vi "Send single trigger.vi"(8 "error in (no error)":errorcluster, 11 "SA-ESA in":refnum<class "SA-ESA.lvclass">) -> (0 "error out":errorcluster, 3 "SA-ESA out":refnum<class "SA-ESA.lvclass">)   [LabVIEW 2020, in "SA-ESA.lvclass"]
uses:
  SA-ESA.lvclass
  C:/Sandbox/RF Bench/Source Code/WiSpry Test Framework/Instruments/Instrument.lvclass
  C:/Sandbox/RF Bench/Source Code/WiSpry Test Framework/Instruments/Spectrum Analyzer/Spectrum Analyzer.lvclass
  Spectrum Analyzer.lvclass/Spectrum Analyzer.ctl
  Instrument.lvclass/Instrument.ctl
  Instrument.lvclass
  Spectrum Analyzer.lvclass
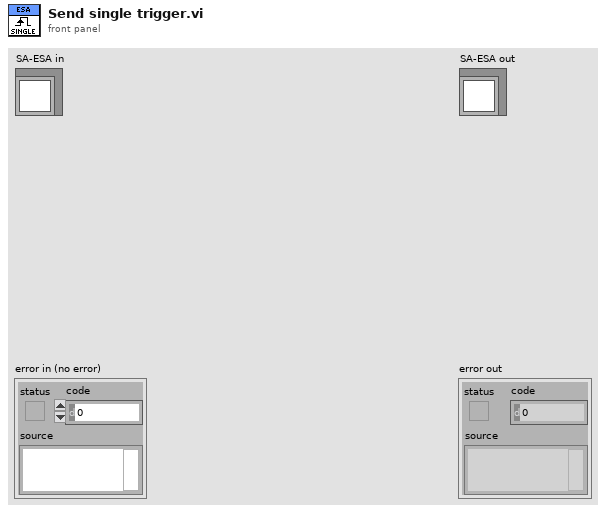
[diagram p1: front panel]
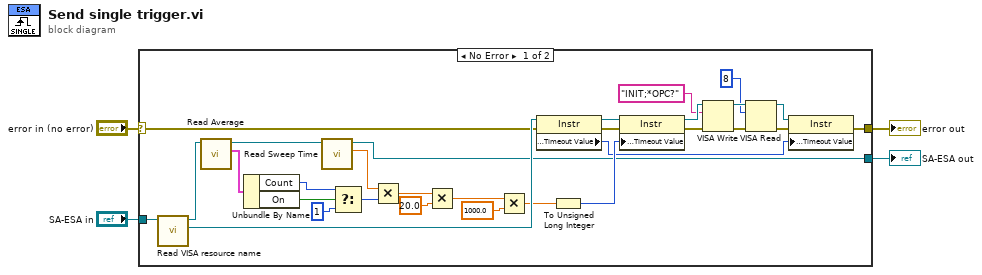
[diagram p0: block diagram]
diagram:
  n1 = case shown="No Error" "error in (no error)" {
    selector: "error in (no error)" -> [w7 w35]
    tunnel: "SA-ESA in" -> [w8 w36]
    tunnel: [w6 w35] -> w2
    tunnel: [w5 w36] -> w1
    frame No Error {
      n2 = call "Read VISA resource name.vi"("Instrument in"=w8) -> ("VISA resource name"=w34:refnum<visa-resource-name>, "Instrument out"=w33:refnum<class "SA-ESA.lvclass">)  [unwired: 9 in]
      n3 = call "Read Average.vi"("Spectrum Analyzer in"=w33) -> ("Average"=w31:cluster{"Count":u32, "On":bool}, "Spectrum Analyzer out"=w32:refnum<class "SA-ESA.lvclass">)  [unwired: 9 in]
      n4 = Unbundle By Name(w31) -> ("Count"=w29:u32, "On"=w30:bool)
      n5 = call "Read Sweep Time.vi"("Spectrum Analyzer in"=w32) -> ("Sweep Time"=w27:dbl, "Spectrum Analyzer out"=w5:refnum<class "SA-ESA.lvclass">)  [unwired: 9 in]
      n6 = Select(t=w29, s=w30, f=u32 1) -> (s? t:f=w26:u32)
      n7 = Multiply(x=w27, y=w26) -> (x*y=w25:dbl)
      n8 = Multiply(x=w25, y=20.0) -> (x*y=w23:dbl)
      n9 = Multiply(x=w23, y=1000.0) -> (x*y=w19:dbl)
      n10 = property class="Instr"(reference=w34, error in=w7) -> (reference out=w21:refnum<visa-resource-name>, error out=w20:errorcluster, "General Settings:Timeout Value"=w9:u32)
      n11 = To Unsigned Long Integer(number=w19) -> (unsigned 32bit integer=w18:u32)
      n12 = property class="Instr"(reference=w21, error in=w20, "General Settings:Timeout Value"=w18) -> (reference out=w17:refnum<visa-resource-name>, error out=w16:errorcluster)
      n13 = VISA Write(VISA resource name=w17, write buffer="INIT;*OPC?", error in (no error)=w16) -> (VISA resource name out=w13:refnum<visa-resource-name>, error out=w14:errorcluster)  [unwired: 1 out]
      n14 = VISA Read(VISA resource name=w13, byte count=u32 8, error in (no error)=w14) -> (VISA resource name out=w11:refnum<visa-resource-name>, error out=w10:errorcluster)  [unwired: 2 out]
      n15 = property class="Instr"(reference=w11, error in=w10, "General Settings:Timeout Value"=w9) -> (error out=w6:errorcluster)  [unwired: 1 out]
    }
    frame Error {
    }
  }
  "error out" <- w2
  "SA-ESA out" <- w1
